vi "Get Resource ID.vi"(4 "SPI CS in":refnum<class "SPI CS.lvclass">) -> (7 "Resource ID":string)   [LabVIEW 2020, in "CTI.lvlib" / "SPI CS.lvclass"]
uses:
  SPI CS.lvclass
  SPI CS.lvclass/SPI CS.ctl
  GPIO/GPIO.lvclass/GPIO.ctl
  GPIO/GPIO.lvclass
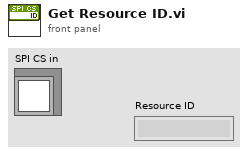
[diagram p1: front panel]
types:
  T1 = typedef "CTI.lvlib/GPIO Number.ctl" = i8
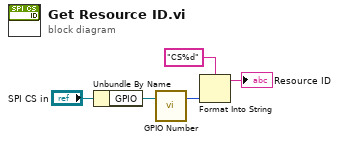
[diagram p0: block diagram]
diagram:
  n1 = Unbundle By Name("SPI CS in") -> ("GPIO"=w4:refnum<class "GPIO.lvclass">)
  n2 = call "GPIO Number.vi"("GPIO in"=w4) -> ("GPIO #"=w3:T1)  [unwired: 6 in]
  n3 = Format Into String(format string="CS%d", w3) -> (resulting string=→"Resource ID":string)  [unwired: 2 in, 1 out]
